vi "ConfigTiming.vi"(8 "error in (no error)":errorcluster, 10 "Wait Time (500 ms)":u32=500, 11 "PXI_MultiTrig in":refnum<class "PXI_MultiTrig.lvclass">) -> (0 "error out":errorcluster, 3 "PXI_MultiTrig out":refnum<class "PXI_MultiTrig.lvclass">)   [LabVIEW 2014, in "SyncPlugins.lvlib" / "PXI_MultiTrig.lvclass"]
uses:
  PXI_MultiTrig.lvclass
  PXI_MultiTrig.lvclass/PXI_MultiTrig.ctl
  SyncPluginBase/SyncPluginBase.lvclass/SyncPluginBase.ctl
  Accessors/Read TimingHandle.vi
  Accessors/Write TimingSession.vi
  SyncPluginBase/Accessors/Write Initiated.vi
  <instrlib>/niSync/niSync.llb/niSync Initialize (IVI).vi
  <vilib>/Utility/error.llb/Error Cluster From Error Code.vi
  <vilib>/ErrorRing/Error Ring.xnode
panel:
  out "Retries":i32
  out "PLL Locked?":bool
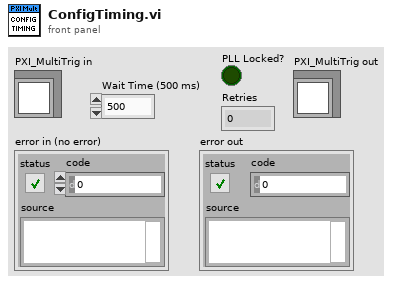
[diagram p1: front panel]
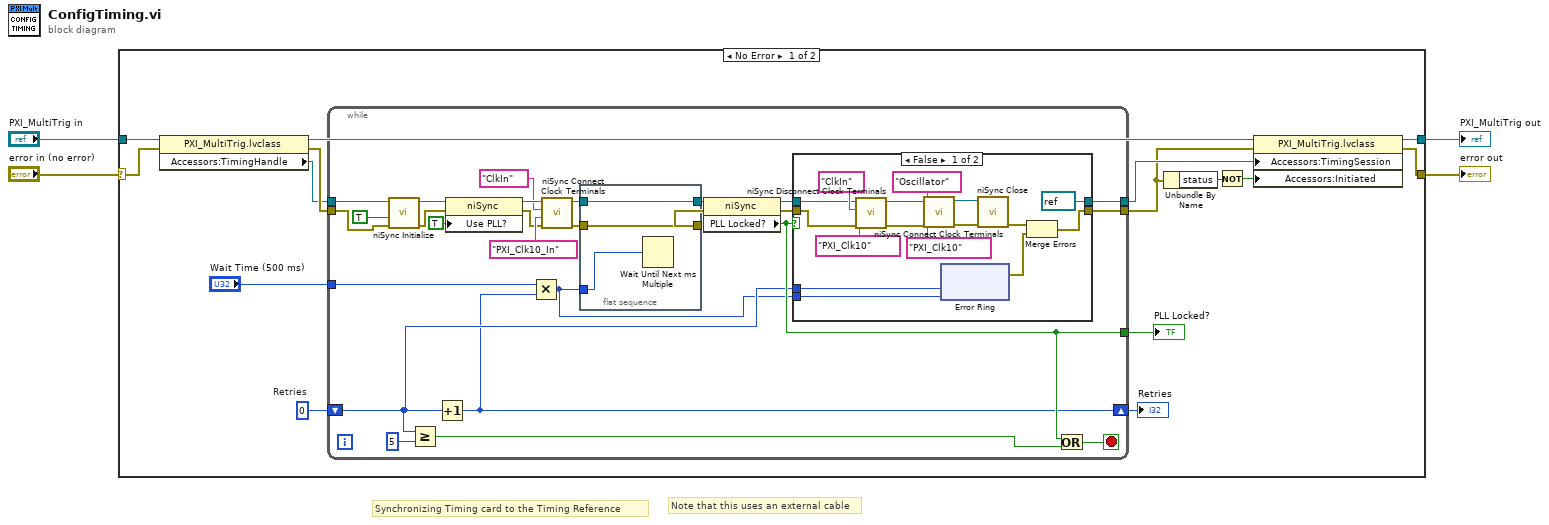
[diagram p0: block diagram]
diagram:
  # "Note that this uses an external cable"
  # "Synchronizing Timing card to the Timing Reference"
  n1 = case shown="No Error" "error in (no error)" {
    selector: "error in (no error)" -> [w14 w75]
    tunnel: [w19 w75] -> w4
    tunnel: [w15 w76] -> w3
    tunnel: "PXI_MultiTrig in" -> [w13 w76]
    frame No Error {
      w8 = 0  # Retries
      n2 = property class="PXI_MultiTrig.lvclass"(reference=w13, error in=w14) -> (reference out=w11:refnum<class "PXI_MultiTrig.lvclass">, error out=w12:errorcluster, "Accessors:TimingHandle"=w10:refnum<k15>)
      n3 = while {
        shift-right: [w22] -> w6
        shift-left: w8 -> [w23]
        tunnel: [w26] -> w7
        tunnel: w12 -> [w44]
        tunnel: [w31] -> w9
        tunnel: "Wait Time (500 ms)" -> [w21]
        tunnel: w10 -> [w32]
        tunnel: [w45] -> w18
        stop <- w27 stop-if-true
        n4 = call-poly <instrlib>:"niSync Initialize.vi"("error in (no error)"=w44, "reset device (F)"=TRUE, "resource name"=w32) -> ("error out"=w30:errorcluster, "instrument handle out"=w33:refnum<k15>)  [unwired: 7 in]
        n5 = Greater Or Equal?(x=w23, y=5) -> (x >= y?=w24:bool)
        n6 = Increment(x=w23) -> (x+1=w22:i32)
        n7 = property class="niSync"(reference=w33, error in=w30, "Use PLL?"=TRUE ("Clk Properties:Use PLL?")) -> (reference out=w36:refnum<k15>, error out=w29:errorcluster)
        n8 = Multiply(x=w21, y=w22) -> (x*y=w20:u32)
        n9 = call <instrlib>:"niSync Connect Clock Terminals.vi"("error in (no error)"=w29, "destination terminal"="PXI_Clk10_In", "source terminal"="ClkIn", "instrument handle"=w36) -> ("error out"=w39:errorcluster, "instrument handle out"=w38:refnum<k15>)  [unwired: 6 in]
        n10 = flat-sequence {
          tunnel: w38 -> [w74]
          tunnel: w39 -> [w73]
          tunnel: [w74] -> w41
          tunnel: [w73] -> w40
          tunnel: w20 -> [w72]
          frame #0 {
            n11 = Wait Until Next ms Multiple(millisecond multiple=w72) -> ()  [unwired: 1 out]
          }
        }
        n12 = property class="niSync"(reference=w41, error in=w40) -> (reference out=w42:refnum<k15>, error out=w43:errorcluster, "PLL Locked?"=w26:bool)
        n13 = case shown="False" w26 {
          tunnel: w42 -> [w57 w71]
          tunnel: w43 -> [w55 w70]
          tunnel: [refnum<k15> refnum ("instrument handle out") w71] -> w45
          tunnel: [w46 w70] -> w31
          tunnel: w23 -> [w49 _]
          tunnel: w20 -> [w48 _]
          frame False {
            n14 = call <instrlib>:"niSync Disconnect Clock Terminals.vi"("error in (no error)"=w55, "destination terminal"="PXI_Clk10", "source terminal"="ClkIn", "instrument handle"=w57) -> ("error out"=w54:errorcluster, "instrument handle out"=w56:refnum<k15>)  [unwired: 6 in]
            n15 = call <instrlib>:"niSync Connect Clock Terminals.vi"("error in (no error)"=w54, "destination terminal"="PXI_Clk10", "source terminal"="Oscillator", "instrument handle"=w56) -> ("error out"=w52:errorcluster, "instrument handle out"=w53:refnum<k15>)  [unwired: 6 in]
            n16 = xnode "Error Ring"("parameter 0"=w49, "parameter 1"=w48) -> ("error out"=w50:errorcluster)
            n17 = call <instrlib>:"niSync Close.vi"("error in (no error)"=w52, "instrument handle"=w53) -> ("error out"=w51:errorcluster)  [unwired: 9 in]
            n18 = Merge Errors(w51, w50) -> (w46:errorcluster)
          }
          frame True {
          }
        }
        n19 = Or(x=w26, y=w24) -> (x .or. y?=w27:bool)
      }
      "PLL Locked?" <- w7
      "Retries" <- w6
      n20 = Unbundle By Name(w9) -> ("status"=w16:bool)
      n21 = Not(x=w16) -> (.not. x?=w17:bool)
      n22 = property class="PXI_MultiTrig.lvclass"(reference=w11, error in=w9, "Accessors:TimingSession"=w18, "Accessors:Initiated"=w17) -> (reference out=w15:refnum<class "PXI_MultiTrig.lvclass">, error out=w19:errorcluster)
    }
    frame Error {
    }
  }
  "error out" <- w4
  "PXI_MultiTrig out" <- w3
